vi "CreatingSubVisSubVi.vi"(1 "Boolean":bool, 2 "Slide":dbl) -> (0 "Numeric":dbl)   [LabVIEW 2018]
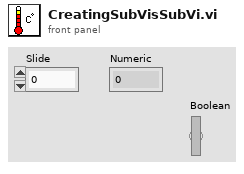
[diagram p1: front panel]
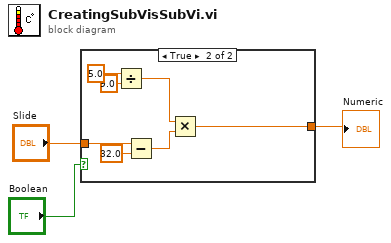
[diagram p0: block diagram]
diagram:
  n1 = case shown="True" "Boolean" {
    tunnel: "Slide" -> [w4 w11]
    tunnel: [w4 w5] -> w1
    frame False {
    }
    frame True {
      n2 = Divide(x=5.0, y=9.0) -> (x/y=w7:dbl)
      n3 = Subtract(x=w11, y=32.0) -> (x-y=w6:dbl)
      n4 = Multiply(x=w7, y=w6) -> (x*y=w5:dbl)
    }
  }
  "Numeric" <- w1
